vi "String Length with math .vi"() -> ()   [LabVIEW 2020]
panel:
  out "SDI":u64[](array[numeric]) format="%.0x"
  out "Result of comparission":string
  out "if false":string
  out "Length in bytes":i32
  out "Array":string[](array[string])
  in  "String":string
  out "SDO":u64[](array[numeric]) format="%.0x"
  out "max(x,y)":i32[](array[numeric])
  out "y":i32
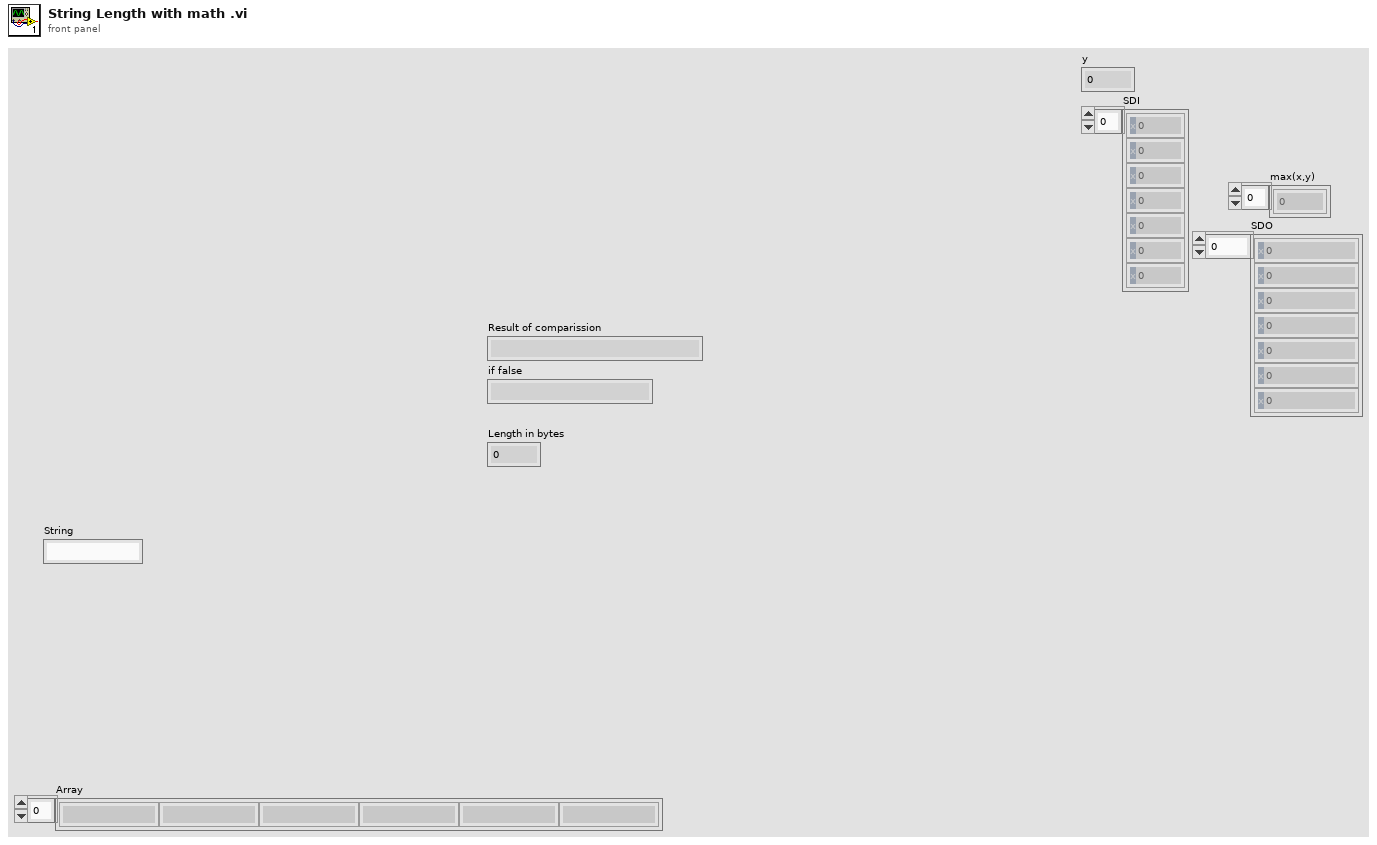
[diagram p1: front panel]
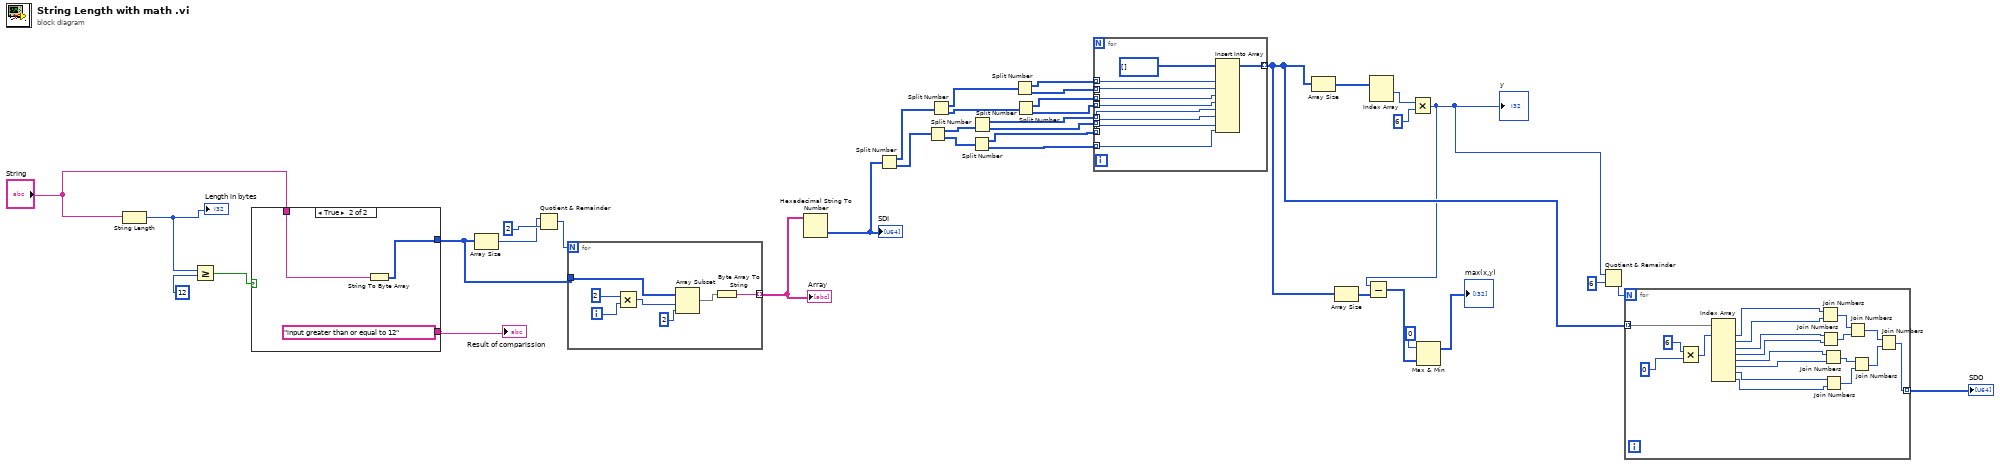
[diagram p0: block diagram]
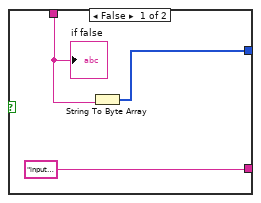
[diagram p2: hidden frame]
diagram:
  n1 = String Length(string="String") -> (length=w4:i32)
  "Length in bytes" <- w4
  n2 = Greater Or Equal?(x=w4, y=12) -> (x >= y?=w8:bool)
  n3 = case shown="True" w8 {
    tunnel: [w38 w43] -> w7
    tunnel: "String" -> [w39 w42]
    tunnel: ["input less than 12" "input greater than or equal to 12"] -> w5
    frame False {
      n4 = String To Byte Array(string=w39) -> (unsigned byte array=w38:u8[])
      "if false" <- w39
    }
    frame True {
      n5 = String To Byte Array(string=w42) -> (unsigned byte array=w43:u8[])
    }
  }
  "Result of comparission" <- w5
  n6 = Array Size(array=w7) -> (size(s)=w2:i32)
  n7 = Quotient & Remainder(x=w2, y=2) -> (floor(x/y)=w11:i32)  [unwired: 1 out]
  n8 = for {
    N: w11 -> [_]
    tunnel: w7 -> [w50]
    tunnel: [w47] -> w10 mode=indexing
    i -> [w45]
    n9 = Multiply(x=2 ("y"), y=w45) -> (x*y=w49:i32)
    n10 = Array Subset(array=w50, index=w49, length=2) -> (w46:u8[])
    n11 = Byte Array To String(unsigned byte array=w46) -> (string=w47:string)
  }
  "Array" <- w10
  n12 = Hexadecimal String To Number(string=w10) -> (number=w1:u32[])  [unwired: 2 in, 1 out]
  "SDI" <- w1
  n13 = Split Number(x=w1) -> (hi(x)=w33:u16[], lo(x)=w34:u16[])
  n14 = Split Number(x=w34) -> (hi(x)=w35:u8[], lo(x)=w28:u8[])
  n15 = Split Number(x=w33) -> (hi(x)=w37:u8[], lo(x)=w36:u8[])
  n16 = Split Number(x=w28) -> (hi(x)=w25:u8[], lo(x)=w24:u8[])
  n17 = Split Number(x=w35) -> (hi(x)=w27:u8[], lo(x)=w26:u8[])
  n18 = Split Number(x=w37) -> (hi(x)=w32:u8[], lo(x)=w31:u8[])
  n19 = Split Number(x=w36) -> (hi(x)=w30:u8[], lo(x)=w29:u8[])
  n20 = for {
    tunnel: [w60] -> w13 mode=indexing
    tunnel: w32 -> [w58] mode=indexing
    tunnel: w31 -> [w57] mode=indexing
    tunnel: w30 -> [w56] mode=indexing
    tunnel: w29 -> [w55] mode=indexing
    tunnel: w27 -> [w54] mode=indexing
    tunnel: w26 -> [w53] mode=indexing
    tunnel: w25 -> [w52] mode=indexing
    tunnel: w24 -> [w51] mode=indexing
    n21 = Insert Into Array(array=u8[] [], new element #1=w58, new element #2=w57, new element #3=w56, new element #4=w55, new element #5=w54, new element #6=w53, new element #7=w52, new element #8=w51) -> (w60:u8[])  [unwired: 1 in]
  }
  n22 = Array Size(array=w13) -> (size(s)=w23:i32[])
  n23 = Array Size(array=w13) -> (size(s)=w17:i32[])
  n24 = Index Array(array=w23) -> (element #1=w22:i32)  [unwired: 2 in, 1 out]
  n25 = Multiply(x=w22, y=6) -> (x*y=w12:i32)
  "y" <- w12
  n26 = Subtract(x=w12, y=w17) -> (x-y=w20:i32[])
  n27 = Max & Min(x=0, y=w20) -> (max(x,y)=→"max(x,y)":i32[])  [unwired: 1 out]
  n28 = Quotient & Remainder(x=w12, y=6) -> (floor(x/y)=w15:i32)  [unwired: 1 out]
  n29 = for {
    N: w15 -> [_]
    tunnel: [w77] -> w14 mode=indexing
    tunnel: w13 -> [w76] mode=indexing
    n30 = Multiply(x=6, y=0) -> (x*y=w78:i32)
    n31 = Index Array(array=w76, index #1=w78) -> (element #1=w69:u8, element #2=w68:u8, element #3=w67:u8, element #4=w66:u8, element #5=w65:u8, element #6=w64:u8, element #7=w63:u8, element #8=w62:u8)  [unwired: 7 in]
    n32 = Join Numbers(hi=w69, lo=w68) -> ((hi.lo)=w71:u16)
    n33 = Join Numbers(hi=w67, lo=w66) -> ((hi.lo)=w70:u16)
    n34 = Join Numbers(hi=w65, lo=w64) -> ((hi.lo)=w73:u16)
    n35 = Join Numbers(hi=w63, lo=w62) -> ((hi.lo)=w72:u16)
    n36 = Join Numbers(hi=w71, lo=w70) -> ((hi.lo)=w75:u32)
    n37 = Join Numbers(hi=w73, lo=w72) -> ((hi.lo)=w74:u32)
    n38 = Join Numbers(hi=w75, lo=w74) -> ((hi.lo)=w77:u64)
  }
  "SDO" <- w14
